vi "Execute.vi"(8 "error in (no error)":errorcluster, 10 "Context in":refnum<class "Context.lvclass">, 11 "Enable Command in":refnum<class "Enable Command.lvclass">) -> (0 "error out":errorcluster, 2 "Context out":refnum<class "Context.lvclass">, 3 "Enable Command out":refnum<class "Enable Command.lvclass">)   [LabVIEW 2015, in "Enable Command.lvclass"]
uses:
  Enable Command.lvclass
  Context/Context.lvclass
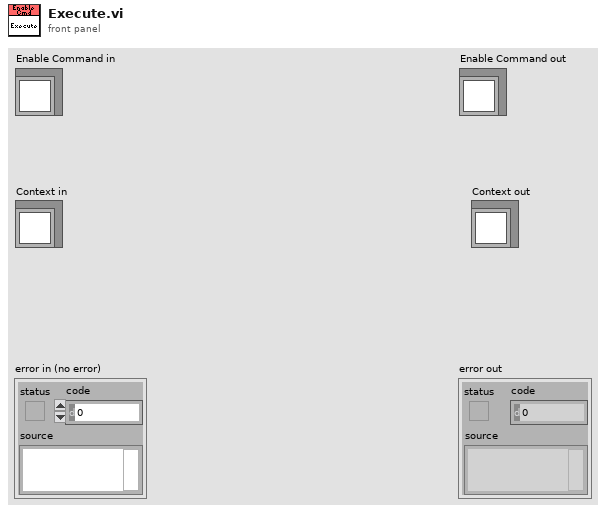
[diagram p1: front panel]
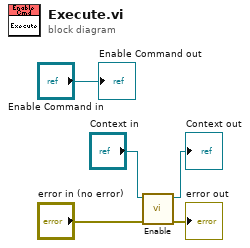
[diagram p0: block diagram]
diagram:
  n1 = call "Enable.vi"("error in (no error)"="error in (no error)", "Context in"="Context in") -> ("error out"=→"error out":errorcluster, "Context out"=→"Context out":refnum<class "Context.lvclass">)  [unwired: 8 in]
  "Enable Command out" <- "Enable Command in"
